vi "Read data value reference.vi"(8 "error in (no error)":errorcluster, 11 "DAQVoltage in":refnum<class "DAQVoltage.lvclass">) -> (0 "error out":errorcluster, 2 "data value reference":refnum<data-value>, 3 "DAQVoltage out":refnum<class "DAQVoltage.lvclass">)   [LabVIEW 2025, in "DAQVoltage.lvlib" / "DAQVoltage.lvclass"]
uses:
  DAQVoltage.lvclass
  DAQVoltage.lvclass/DAQVoltage.ctl
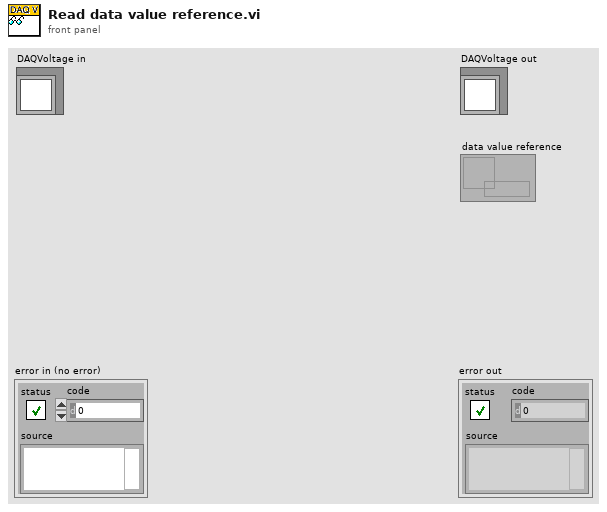
[diagram p1: front panel]
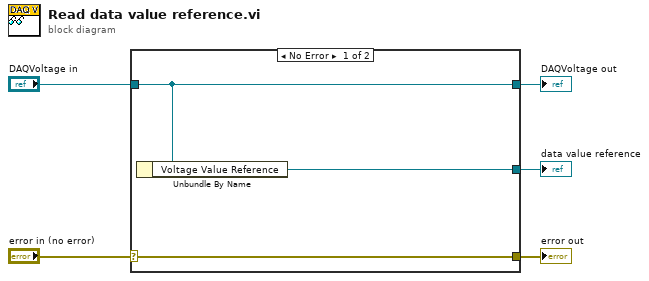
[diagram p0: block diagram]
diagram:
  n1 = case shown="No Error" "error in (no error)" {
    selector: "error in (no error)" -> [w8 w9]
    tunnel: [w8 w9] -> w4
    tunnel: [w7 w10] -> w2
    tunnel: "DAQVoltage in" -> [w7 w10]
    tunnel: [w6 _] -> w1
    frame No Error {
      n2 = Unbundle By Name(w7) -> ("Voltage Value Reference"=w6:refnum<data-value>)
    }
    frame Error {
    }
  }
  "error out" <- w4
  "DAQVoltage out" <- w2
  "data value reference" <- w1
